vi "界面切换.vi"(8 "界面切换队列输入":refnum<queue>, 9 "切换界面名称输入":string, 10 "Bool引用句柄":refnum<vi>, 11 "状态转移输入":refnum<queue>) -> (3 "布尔":bool)   [LabVIEW 2018]
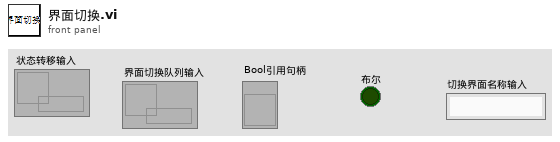
[diagram p1: front panel]
types:
  T1 = enum8{"Enabled", "Disabled", "Disabled and Grayed Out"}
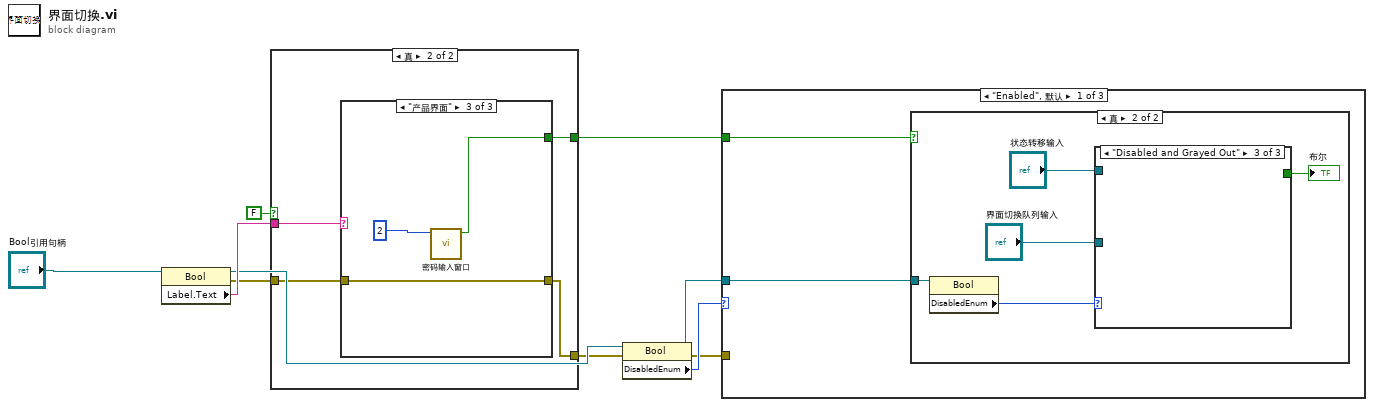
[diagram p0: block diagram]
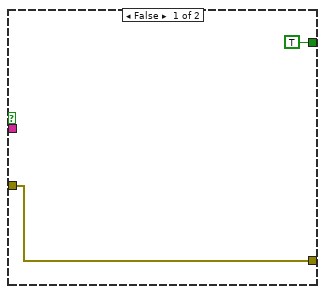
[diagram p2: hidden frame]
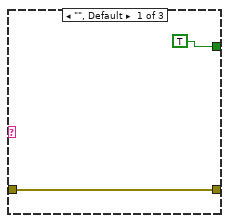
[diagram p3: hidden frame]
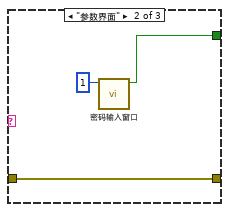
[diagram p4: hidden frame]
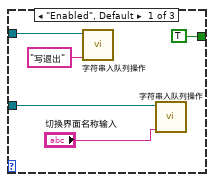
[diagram p6: hidden frame]
diagram:
  n1 = property class="Bool"(reference="Bool引用句柄") -> (reference out=w5:refnum<vi>, error out=w4:errorcluster, "Label.Text"=w6:string)  [unwired: 1 in]
  n2 = case shown="真" FALSE {
    tunnel: [TRUE ("结果") w16] -> w10
    tunnel: w6 -> [_ w15]
    tunnel: w4 -> [w11 w14]
    tunnel: [w11 w13] -> w3
    frame False {
    }
    frame True {
      n3 = case shown="\"产品界面\"" w15 {
        tunnel: [TRUE w20 w23] -> w16
        tunnel: w14 -> [w17 w19 w22]
        tunnel: [w17 w19 w22] -> w13
        frame "", Default {
        }
        frame "参数界面" {
          n4 = call "密码输入窗口.vi"("权限等级"=1) -> ("结果"=w20:bool)  [unwired: 10 in]
        }
        frame "产品界面" {
          n5 = call "密码输入窗口.vi"("权限等级"=2) -> ("结果"=w23:bool)  [unwired: 10 in]
        }
      }
    }
  }
  n6 = property class="Bool"(reference=w5, error in=w3) -> (reference out=w8:refnum<vi>, error out=w2:errorcluster, "DisabledEnum"=w9:T1)
  n7 = case shown="\"Enabled\", 默认" w9 {
    tunnel: w8 -> [w26 _ _]
    tunnel: w10 -> [w25 _ _]
    tunnel: w2 -> [_ _ _]
    frame "Enabled", Default {
      n8 = case shown="真" w25 {
        tunnel: w26 -> [_ w27]
        frame False {
        }
        frame True {
          n9 = property class="Bool"(reference=w27) -> ("DisabledEnum"=w31:T1)  [unwired: 1 in, 2 out]
          n10 = case shown="\"Disabled and Grayed Out\"" w31 {
            tunnel: "状态转移输入" -> [w34 _ _]
            tunnel: "界面切换队列输入" -> [w35 _ _]
            tunnel: [TRUE _ _] -> w30
            frame "Enabled", Default {
              n11 = call "字符串入队列操作.vi"("字符消息入队列"="写退出", "界面切换队列"=w34) -> ()  [unwired: 9 in, 1 out]
              n12 = call "字符串入队列操作.vi"("字符消息入队列"="切换界面名称输入", "界面切换队列"=w35) -> ()  [unwired: 9 in, 1 out]
            }
            frame "Disabled" {
            }
            frame "Disabled and Grayed Out" {
            }
          }
          "布尔" <- w30
        }
      }
    }
    frame "Disabled" {
    }
    frame "Disabled and Grayed Out" {
    }
  }
